vi "Configure Measurement.vi"(6 "Manual Range (1)":dbl=1.0, 7 "Manual Resolution (5.5 Digits)":dbl(ring)=5.5 items=["3.5"=3.5, "4.5"=4.5, "5.5"=5.5], 8 "error in (no error)":errorcluster, 9 "Enable Auto Range (T:Enable)":bool=TRUE, 10 "Function (0: DC Volts)":i32(ring) items=["DC Volts", "AC Volts", "DC Current", "AC Current", "2-Wire Resistance", "Frequency", "Temperature", "Capacitance", "Continuity", "Diode", "4-Wire Resistance", "2nd DC Volts", "2nd AC Volts", "2nd DC Current", "2nd AC Current", "2nd Frequency"], 11 "VISA resource name":refnum<visa-resource-name>) -> (0 "error out":errorcluster, 3 "VISA resource name out":refnum<visa-resource-name>)   [LabVIEW 2020, in "Agilent 34405.lvlib"]
doc: "Configures the measurement type, resolution, and range on the instrument."
uses:
  <instrlib>/Agilent 34405/Agilent 34405.lvlib
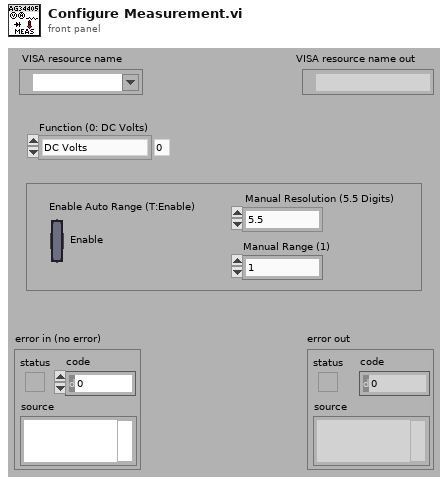
[diagram p1: front panel]
types:
  T1 = typedef "Agilent 34405.lvlib/Extended User Data.ctl" = cluster{"344XX Mode":u16, "Measurement Type":u16}
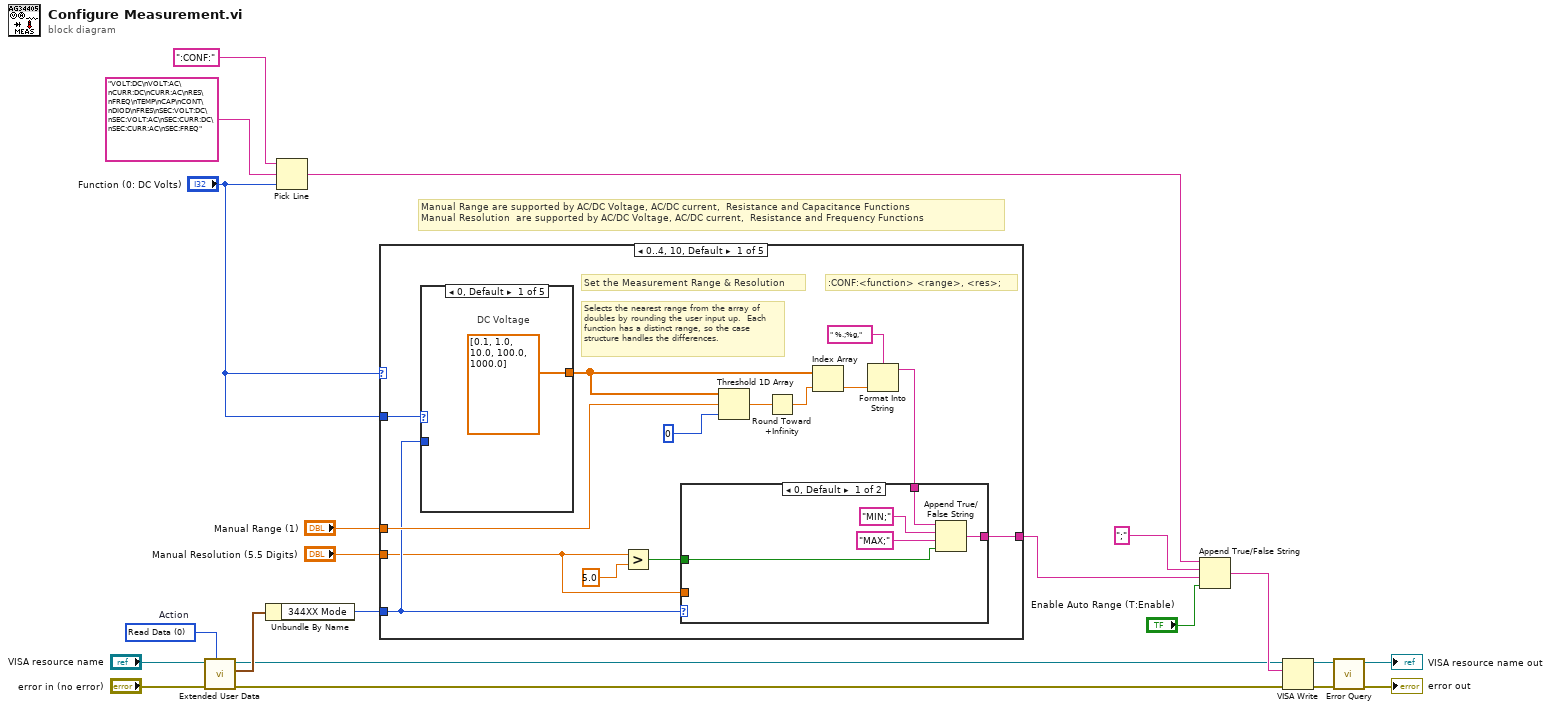
[diagram p0: block diagram]
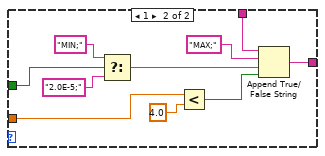
[diagram p2: hidden frame]
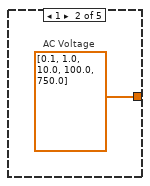
[diagram p3: hidden frame]
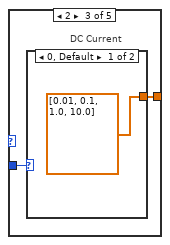
[diagram p4: hidden frame]
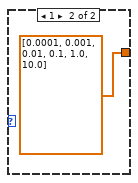
[diagram p5: hidden frame]
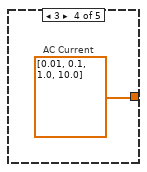
[diagram p6: hidden frame]
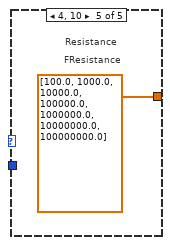
[diagram p7: hidden frame]
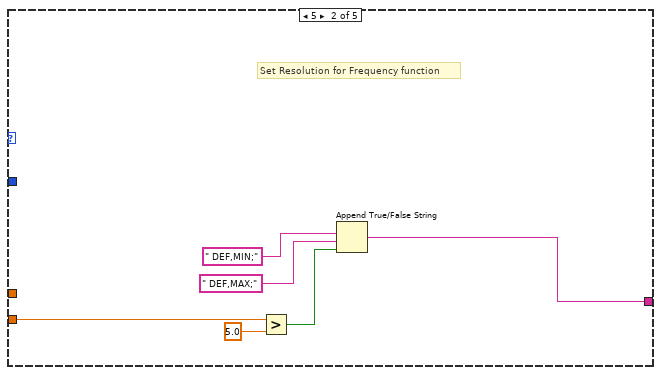
[diagram p8: hidden frame]
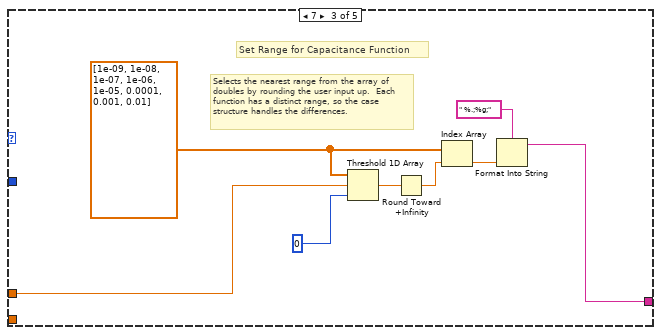
[diagram p9: hidden frame]
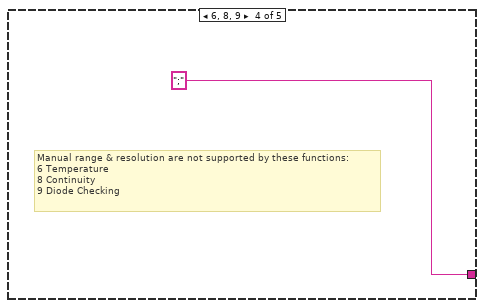
[diagram p10: hidden frame]
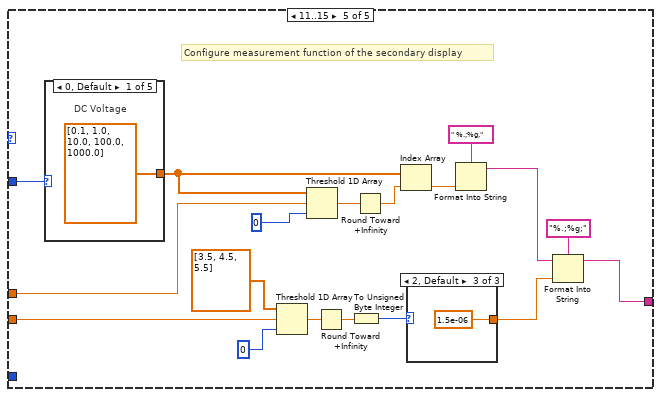
[diagram p11: hidden frame]
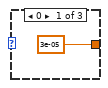
[diagram p12: hidden frame]
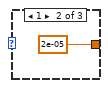
[diagram p13: hidden frame]
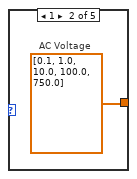
[diagram p14: hidden frame]
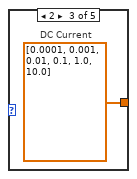
[diagram p15: hidden frame]
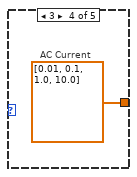
[diagram p16: hidden frame]
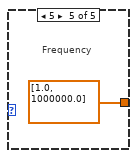
[diagram p17: hidden frame]
diagram:
  w7 = 0 items=["Read Data", "Write Data", "Clear Data", "Clear ALL Data"]  # Action
  # "Manual Range are supported by AC/DC Voltage, AC/DC current,  Resistance and Capacitance Functions\nManual Resolution  are supported by AC/DC Voltage, AC/DC current,  Resistance and Frequency Functions"
  n1 = call <instrlib>:"Extended User Data.vi"("Action"=w7, "error in (no error)"="error in (no error)", "VISA resource name in"="VISA resource name") -> ("error out"=w3:errorcluster, "User Data Out"=w6:T1, "VISA resource name out"=w4:refnum<visa-resource-name>)  [unwired: 1 in, 5 out]
  n2 = Unbundle By Name(w6) -> ("344XX Mode"=w5:u16)
  n3 = Pick Line(string ("")=":CONF:", multi-line string="VOLT:DC\nVOLT:AC\nCURR:DC\nCURR:AC\nRES\nFREQ\nTEMP\nCAP\nCONT\nDIOD\nFRES\nSEC:VOLT:DC\nSEC:VOLT:AC\nSEC:CURR:DC\nSEC:CURR:AC\nSEC:FREQ" ("Function"), line index="Function (0: DC Volts)") -> (output string=w13:string)
  n4 = case shown="0..4, 10, Default" "Function (0: DC Volts)" {
    tunnel: "Function (0: DC Volts)" -> [w28 _ _ _ w81]
    tunnel: [w26 w59 w65 ";" ("Auto Range") w82] -> w2
    tunnel: "Manual Resolution (5.5 Digits)" -> [w22 w60 _ _ w79]
    tunnel: "Manual Range (1)" -> [w29 _ w66 _ w83]
    tunnel: w5 -> [w25 _ _ _ _]
    frame 0..4, 10, Default {
      # "Set the Measurement Range & Resolution"
      # ":CONF:<function> <range>, <res>;"
      # "Selects the nearest range from the array of doubles by rounding the user input up.  Each function has a distinct range, so the case structure handles the differences."
      n5 = case shown="0, Default" w28 {
        tunnel: [dbl[] [0.1, 1.0, 10.0, 100.0, 1000.0] ("Array Constant") dbl[] [0.1, 1.0, 10.0, 100.0, 750.0] ("Array Constant") w54 dbl[] [0.01, 0.1, 1.0, 10.0] ("Array Constant") dbl[] [100.0, 1000.0, 10000.0, 100000.0, 1000000.0, 10000000.0, 100000000.0] ("Array Constant")] -> w31
        tunnel: w25 -> [_ _ w53 _ _]
        frame 0, Default {
          # "DC Voltage"
        }
        frame 1 {
          # "AC Voltage"
        }
        frame 2 {
          # "DC Current"
          n6 = case shown="0, Default" w53 {
            tunnel: [dbl[] [0.01, 0.1, 1.0, 10.0] ("Array Constant") dbl[] [0.0001, 0.001, 0.01, 0.1, 1.0, 10.0] ("Array Constant")] -> w54
            frame 0, Default {
            }
            frame 1 {
            }
          }
        }
        frame 3 {
          # "AC Current"
        }
        frame 4, 10 {
          # "FResistance"
          # "Resistance"
        }
      }
      n7 = Greater?(x=w22, y=5.0) -> (0:w23:bool)
      n8 = Threshold 1D Array(1:0 ("start index (0)"), 2:w29, 3:w31) -> (0:w32:dbl)
      n9 = Round Toward +Infinity ("Round To +Infinity")(x=w32) -> (ceil(x): smallest int >= x=w33:dbl)
      n10 = Index Array(array=w31, index=w33) -> (element=w30:dbl)
      n11 = Format Into String(format string=" %.;%g,", w30) -> (resulting string=w27:string)  [unwired: 2 in, 1 out]
      n12 = case shown="0, Default" w25 {
        tunnel: w27 -> [w38 w43]
        tunnel: [w37 w44] -> w26
        tunnel: w23 -> [w36 w47]
        tunnel: w22 -> [_ w41]
        frame 0, Default {
          n13 = Append True/False String(1:w36, 2:"MAX;" ("false string"), 3:"MIN;" ("true string"), 4:w38) -> (0:w37:string)
        }
        frame 1 {
          n14 = Select(t="MIN;", s=w47, f="2.0E-5;") -> (s? t:f=w45:string)
          n15 = Less?(x=w41, y=4.0) -> (x < y?=w46:bool)
          n16 = Append True/False String(1:w46, 2:w45, 3:"MAX;", 4:w43) -> (0:w44:string)
        }
      }
    }
    frame 5 {
      # "Set Resolution for Frequency function"
      n17 = Greater?(x=w60, y=5.0) -> (0:w61:bool)
      n18 = Append True/False String(1:w61, 2:" DEF,MAX;" ("false string"), 3:" DEF,MIN;" ("true string")) -> (0:w59:string)  [unwired: 1 out]
    }
    frame 7 {
      w68 = dbl[] [1e-09, 1e-08, 1e-07, 1e-06, 1e-05, 0.0001, 0.001, 0.01] ("Array Constant")
      # "Set Range for Capacitance Function"
      # "Selects the nearest range from the array of doubles by rounding the user input up.  Each function has a distinct range, so the case structure handles the differences."
      n19 = Threshold 1D Array(1:0 ("start index (0)"), 2:w66, 3:w68) -> (0:w69:dbl)
      n20 = Round Toward +Infinity ("Round To +Infinity")(x=w69) -> (ceil(x): smallest int >= x=w70:dbl)
      n21 = Index Array(array=w68, index=w70) -> (element=w67:dbl)
      n22 = Format Into String(format string=" %.;%g;", w67) -> (resulting string=w65:string)  [unwired: 2 in, 1 out]
    }
    frame 6, 8, 9 {
      # "Manual range & resolution are not supported by these functions:\n6 Temperature\n8 Continuity\n9 Diode Checking"
    }
    frame 11..15 {
      # "Configure measurement function of the secondary display"
      n23 = case shown="0, Default" w81 {
        tunnel: [dbl[] [0.1, 1.0, 10.0, 100.0, 1000.0] ("Array Constant") dbl[] [0.1, 1.0, 10.0, 100.0, 750.0] ("Array Constant") dbl[] [0.0001, 0.001, 0.01, 0.1, 1.0, 10.0] ("Array Constant") dbl[] [0.01, 0.1, 1.0, 10.0] ("Array Constant") dbl[] [1.0, 1000000.0] ("Array Constant")] -> w89
        frame 0, Default {
          # "DC Voltage"
        }
        frame 1 {
          # "AC Voltage"
        }
        frame 2 {
          # "DC Current"
        }
        frame 3 {
          # "AC Current"
        }
        frame 5 {
          # "Frequency"
        }
      }
      n24 = Threshold 1D Array(1:0 ("start index (0)"), 2:w79, 3:dbl[] [3.5, 4.5, 5.5] ("Array Constant")) -> (0:w77:dbl)
      n25 = Threshold 1D Array(1:0 ("start index (0)"), 2:w83, 3:w89) -> (0:w87:dbl)
      n26 = Round Toward +Infinity ("Round To +Infinity")(x=w77) -> (ceil(x): smallest int >= x=w76:dbl)
      n27 = To Unsigned Byte Integer(number=w76) -> (unsigned 8bit integer=w75:u8)
      n28 = Round Toward +Infinity ("Round To +Infinity")(x=w87) -> (ceil(x): smallest int >= x=w86:dbl)
      n29 = Index Array(array=w89, index=w86) -> (element=w88:dbl)
      n30 = case shown="2, Default" w75 {
        tunnel: [3e-05 2e-05 1.5e-06] -> w74
        frame 0 {
        }
        frame 1 {
        }
        frame 2, Default {
        }
      }
      n31 = Format Into String(format string=" %.;%g,", w88) -> (resulting string=w90:string)  [unwired: 2 in, 1 out]
      n32 = Format Into String(format string="%.;%g;", initial string=w90, w74) -> (resulting string=w82:string)  [unwired: 1 in, 1 out]
    }
  }
  n33 = Append True/False String(1:"Enable Auto Range (T:Enable)", 2:w2, 3:";" ("true string"), 4:w13) -> (0:w11:string)
  n34 = VISA Write(VISA resource name=w4, write buffer=w11, error in (no error)=w3) -> (VISA resource name out=w18:refnum<visa-resource-name>, error out=w17:errorcluster)  [unwired: 1 out]
  n35 = call <instrlib>:"Error Query.vi"("error in (no error)"=w17, "VISA resource name"=w18) -> ("error out"=→"error out":errorcluster, "VISA resource name out"=→"VISA resource name out":refnum<visa-resource-name>)  [unwired: 8 out]
